vi "Initialize UUT States.vi"(8 "error in (no error)":errorcluster, 10 "Number of UUTs":u32, 11 "Example Application in":refnum<class "Example Application.lvclass">) -> (0 "error out":errorcluster, 3 "Example Application out":refnum<class "Example Application.lvclass">)   [LabVIEW 2015, in "Example Application.lvlib" / "Example Application.lvclass"]
uses:
  Example Application.lvclass
  Properties/DUT State -- Enum.ctl
  Example Application.lvclass/Example Application.ctl
  Properties/Example App Properties.lvclass
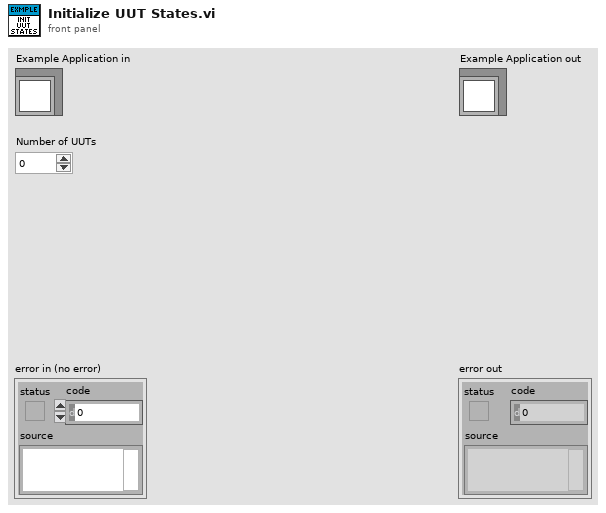
[diagram p1: front panel]
types:
  T1 = typedef "Example Application.lvlib/Example App Properties.lvclass/DUT State -- Enum.ctl" = enum16{"Idle", "Ready", "Testing", "Passed", "Failed"}
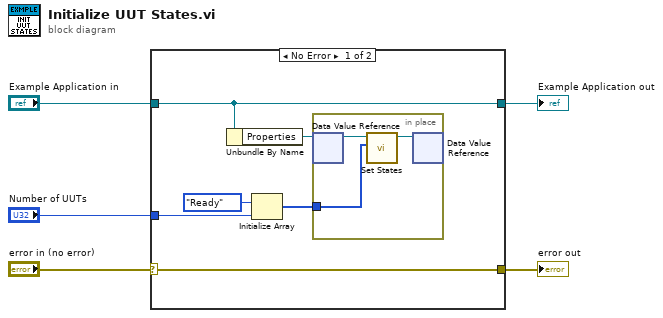
[diagram p0: block diagram]
diagram:
  n1 = case shown="No Error" "error in (no error)" {
    selector: "error in (no error)" -> [w6 w15]
    tunnel: "Example Application in" -> [w10 w16]
    tunnel: "Number of UUTs" -> [w9 _]
    tunnel: [w10 w16] -> w2
    tunnel: [w6 w15] -> w1
    frame No Error {
      n2 = Unbundle By Name(w10) -> ("Properties"=w11:refnum<data-value>)
      n3 = Initialize Array(DUT_State_--_Enum."Ready" ("Enum"), w9) -> (w7:T1[])
      n4 = in-place {
        in-place-border: w7 -> [w12]
        n5 = in-place-dvr #1(w11) -> (w14:refnum<class "Example App Properties.lvclass">)  [unwired: 1 out]
        n6 = call-dynamic "Set States.vi"("UUT States"=w12, "Example App Properties in"=w14) -> ("Example App Properties out"=w13:refnum<class "Example App Properties.lvclass">)  [unwired: 8 in, 1 out]
        n7 = in-place-dvr #1(w13) -> ()  [unwired: 2 out]
      }
    }
    frame Error {
    }
  }
  "error out" <- w1
  "Example Application out" <- w2
